vi "PantherLAB_Log - Add New DQMH Module.vi"(4 "New Module Name":string, 6 "New Module Folder":path, 9 "External Module Info":T1, 10 "New Module Type":T3, 11 "Project":refnum<vi>) -> (0 "error out":errorcluster)   [LabVIEW 2016]
doc: "_____\nCreated using DQMH Framework: Event Scripter 7.1.0.1450."
uses:
  <vilib>/Delacor/Delacor QMH/Libraries/_Scripting Support/Module Type (Including External)--enum.ctl
  <vilib>/Delacor/Delacor QMH/Libraries/_Scripting Support/External Module Info--cluster.ctl
  <vilib>/Delacor/Delacor QMH/Libraries/_Scripting Support/Module Type--enum.ctl
  PantherLAB Scripting Hooks/PantherLAB_Scripting.lvlib
  <vilib>/Delacor/Delacor QMH/Libraries/_Scripting Support/dqmh_lib_DQMH Scripting Support.lvlib
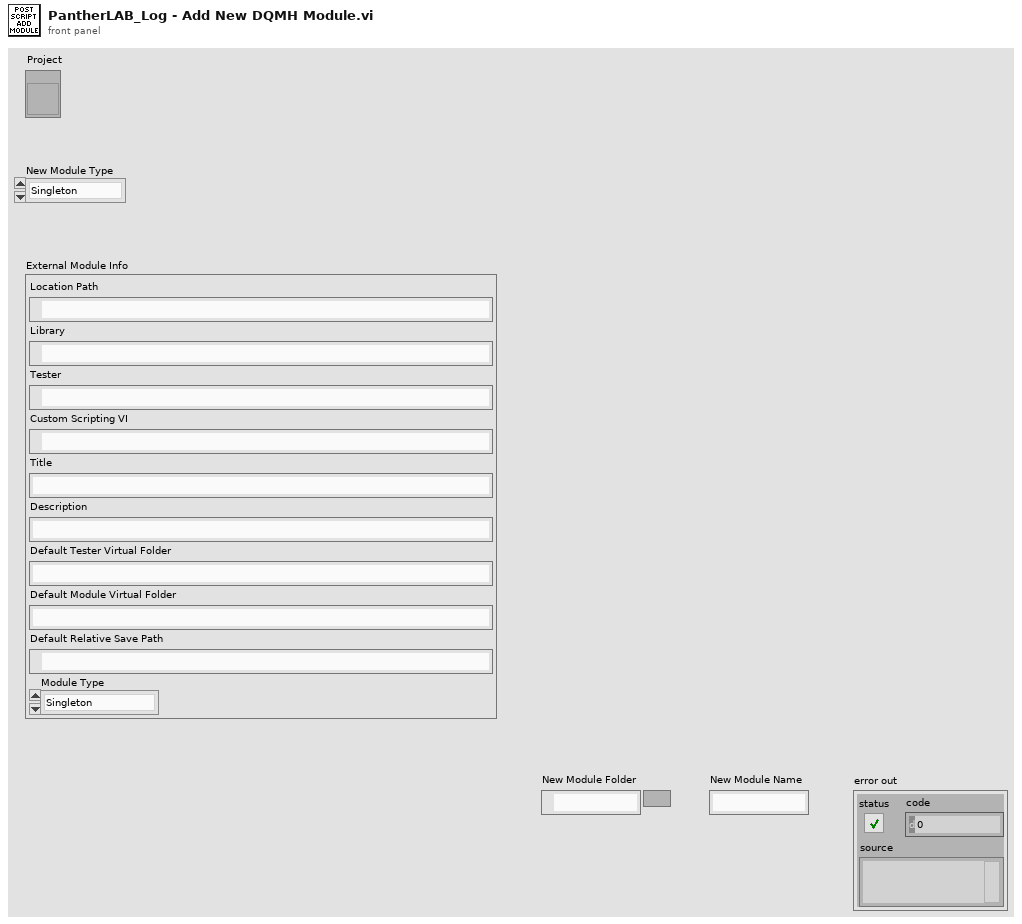
[diagram p1: front panel]
types:
  T1 = typedef "dqmh_lib_DQMH Scripting Support.lvlib/External Module Info--cluster.ctl" = cluster{"Location Path":path, "Library":path, "Tester":path, "Custom Scripting VI":path, "Title":string, "Description":string, "Default Tester Virtual Folder":string, "Default Module Virtual Folder":string, "Default Relative Save Path":path, "Module Type":T2}
  T2 = typedef "dqmh_lib_DQMH Scripting Support.lvlib/Module Type--enum.ctl" = enum16{"Singleton", "Cloneable"}
  T3 = typedef "dqmh_lib_DQMH Scripting Support.lvlib/Module Type (Including External)--enum.ctl" = enum16{"Singleton", "Cloneable", "External"}
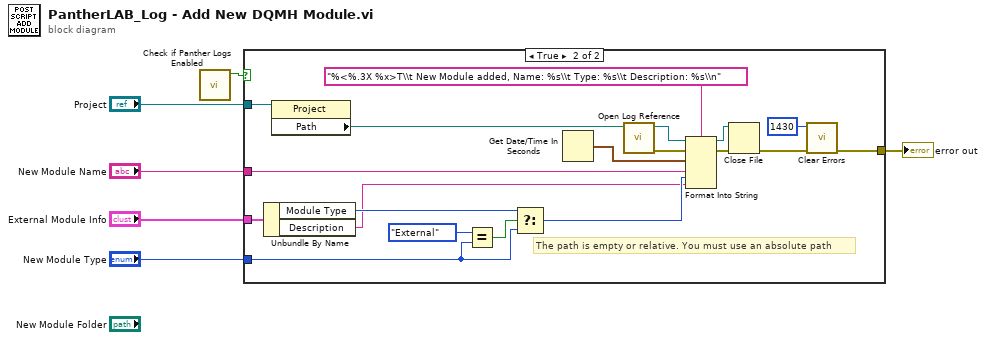
[diagram p0: block diagram]
diagram:
  n1 = call "Check if Panther Logs Enabled.vi"() -> ("PantherLogs Enabled?"=w5:bool)  [unwired: 11 in]
  n2 = case shown="True" w5 {
    tunnel: [_ w8] -> w6
    tunnel: "Project" -> [_ w18]
    tunnel: "New Module Type" -> [_ w11]
    tunnel: "New Module Name" -> [_ w17]
    tunnel: "External Module Info" -> [_ w15]
    frame False {
    }
    frame True {
      # "The path is empty or relative. You must use an absolute path"
      n3 = Unbundle By Name(w15) -> ("Module Type"=w12:T2, "Description"=w9:string)
      n4 = property class="Project"(reference=w18) -> ("Path"=w19:path)  [unwired: 1 in, 2 out]
      n5 = Equal?(x=Module_Type_(Including_External)--enum."External" ("y"), y=w11) -> (x = y?=w14:bool)
      n6 = Select(t=w12, s=w14, f=w11) -> (s? t:f=w10:T3)
      n7 = Get Date/Time In Seconds() -> (seconds since 1Jan1904=w20:timestamp)
      n8 = call "Open Log Reference.vi"("Project Path"=w19) -> ("error out"=w25:errorcluster, "File Reference"=w22:refnum<file>)  [unwired: 9 in]
      n9 = Format Into String(format string="%<%.3X %x>T\\t New Module added, Name: %s\\t Type: %s\\t Description: %s\\n", initial string=w22, error in=w25, w20, w17, w10, w9) -> (resulting string=w21:refnum<file>, error out=w24:errorcluster)
      n10 = Close File(refnum=w21, error in=w24) -> (error out=w23:errorcluster)  [unwired: 1 out]
      n11 = call <vilib>:"Clear Errors.vi"("error in (no error)"=w23, "specific error code to clear (0: all)"=1430) -> ("error out"=w8:errorcluster)  [unwired: 4 in, 1 out]
    }
  }
  "error out" <- w6
